vi "Intake State Controller.vi"(0 "Intake State":enum16{"Cone", "Cube", "Cube Handoff", "Stow"}(ring)=enum."Stow") -> ()   [LabVIEW 2020]
uses:
  <vilib>/Rock Robotics/WPI/Solenoid/WPI_SolenoidValue.ctl
  <vilib>/Rock Robotics/WPI/ThirdParty/REV Robotics/REVLib/Typedef/Spark MAX Control Type.ctl
  <vilib>/Rock Robotics/WPI/Solenoid/WPI_SolenoidSetEnum.vi
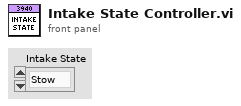
[diagram p1: front panel]
types:
  T1 = typedef "WPI_SolenoidDevRef.ctl" = cluster{"DevStatus":errorcluster, "Pneumatics Control Module":u8, "Forward Solenoid Channel":T2, "Reverse Solenoid Channel":T2}
  T2 = typedef "WPI_SolenoidChannel.ctl" = enum8{"Solenoid 0", "Solenoid 1", "Solenoid 2", "Solenoid 3", "Solenoid 4", "Solenoid 5", "Solenoid 6", "Solenoid 7", "Solenoid 8", "Solenoid 9", "Solenoid 10", "Solenoid 11", "Solenoid 12", "Solenoid 13", "Solenoid 14", "Solenoid 15", "Invalid"}
  T3 = typedef "WPI_MotorControlDeviceRef.ctl" = cluster{"DeviceStatus":errorcluster, "Type":T4, "PWM":cluster{"PWM Channel":T5, "DeadBand":T6}, "CAN":cluster{"Device Number":u8, "SetOutput VI Ref":variant, "GetOutput VI Ref":variant, "Enable VI Ref":variant, "Disable VI Ref":variant, "Data":variant}, "Invert":bool, "DIO PWM":cluster{"PWM \"Enable\" Channel":T5, "DIOChannel":T7, "PWM Rate":dbl}}
  T4 = typedef "WPI_MotorControlType.ctl" = enum16{"PWM", "CAN", "DIO PWM"}
  T5 = typedef "FPGA_DIOPWMChannel.ctl" = enum8{"PWM 0", "PWM 1", "PWM 2", "PWM 3", "PWM 4", "PWM 5", "PWM 6", "PWM 7", "PWM 8", "PWM 9", "PWM MXP 0", "PWM MXP 1", "PWM MXP 2", "PWM MXP 3", "PWM MXP 4", "PWM MXP 5", "PWM MXP 6", "PWM MXP 7", "PWM MXP 8", "PWM MXP 9", "Invalid"}
  T6 = typedef "WPI_PWMDeadband.ctl" = cluster{"Name":string, "maxPositivePwm":i32, "minPositivePwm":i32, "centerPwm":i32, "maxNegativePwm":i32, "minNegativePwm":i32, "angularRange":u16}
  T7 = typedef "FPGA_DIOChannel.ctl" = enum8{"DIO 0", "DIO 1", "DIO 2", "DIO 3", "DIO 4", "DIO 5", "DIO 6", "DIO 7", "DIO 8", "DIO 9", "DIO MXP 0", "DIO MXP 1", "DIO MXP 2", "DIO MXP 3", "DIO MXP 4", "DIO MXP 5", "DIO MXP 6", "DIO MXP 7", "DIO MXP 8", "DIO MXP 9", "DIO MXP 10", "DIO MXP 11", "DIO MXP 12", "DIO MXP 13", "DIO MXP 14", "DIO MXP 15", "SPI Port CS1", "SPI Port CS2", "SPI Port CS3", "SPI Port MISO", "SPI Port MOSI", "Invalid"}
  T8 = typedef "WPI_SolenoidValue.ctl" = enum16{"Off", "On", "Forward", "Reverse"}
  T9 = typedef "Spark MAX Control Type.ctl" = enum16{"Percent VBus", "Voltage", "Velocity", "Position", "Smart Motion", "Current", "Smart Velocity"}
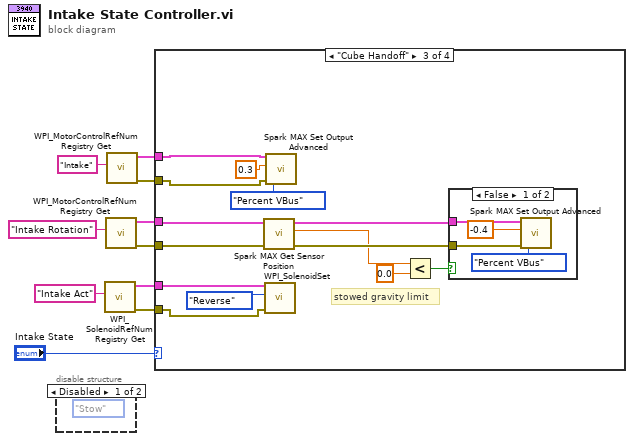
[diagram p0: block diagram]
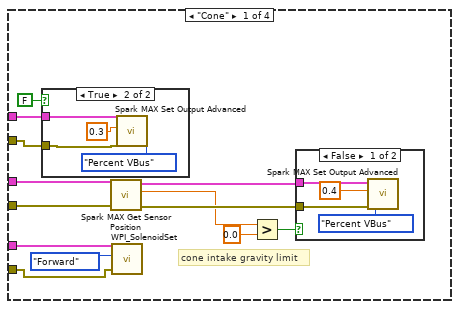
[diagram p3: hidden frame]
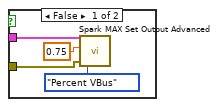
[diagram p4: hidden frame]
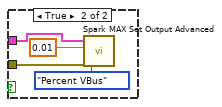
[diagram p5: hidden frame]
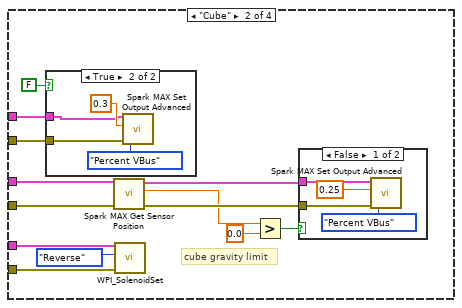
[diagram p6: hidden frame]
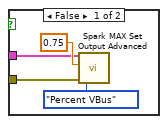
[diagram p7: hidden frame]
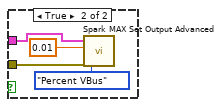
[diagram p8: hidden frame]
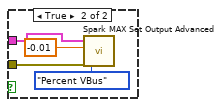
[diagram p9: hidden frame]
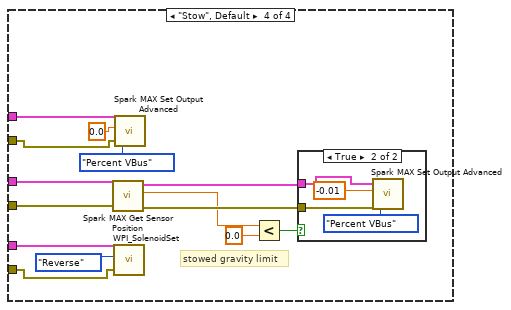
[diagram p10: hidden frame]
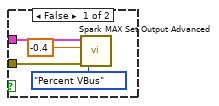
[diagram p11: hidden frame]
diagram:
  n1 = disable-structure shown="Disabled" {
    frame Disabled {
      (unwired) enum16{"Cone", "Cube", "Cube Handoff", "Stow"}."Stow"
    }
    frame Enabled {
    }
  }
  n2 = call <vilib>:"WPI_SolenoidRefNum Registry Get.vi"("refnum name"="Intake Act") -> ("error out"=w9:errorcluster, "SolenoidDevRef"=w10:T1)  [unwired: 9 in]
  n3 = call <vilib>:"WPI_MotorControlRefNum Registry Get.vi"("refnum name"="Intake Rotation") -> ("error out"=w5:errorcluster, "MotorControlDevRef"=w6:T3)  [unwired: 9 in]
  n4 = call <vilib>:"WPI_MotorControlRefNum Registry Get.vi"("refnum name"="Intake") -> ("error out"=w3:errorcluster, "MotorControlDevRef"=w4:T3)  [unwired: 9 in]
  n5 = case shown="\"Cube Handoff\"" "Intake State" {
    tunnel: w10 -> [w17 w42 w78 w92]
    tunnel: w9 -> [w16 w41 w77 w91]
    tunnel: w6 -> [w14 w44 w74 w94]
    tunnel: w5 -> [w15 w43 w73 w93]
    tunnel: w4 -> [w13 w46 w79 w96]
    tunnel: w3 -> [w12 w45 w69 w95]
    frame "Cone" {
      # "cone intake gravity limit"
      n6 = case shown="True" FALSE {
        tunnel: w13 -> [w25 w30]
        tunnel: w12 -> [w24 w29]
        frame False {
          n7 = call <vilib>:"Spark MAX Set Output Advanced.vi"("error in (no error)"=w24, "Control Mode"=Spark_MAX_Control_Type."Percent VBus", "Setpoint"=0.75, "MotorControlDevRef"=w25) -> ()  [unwired: 6 in, 2 out]
        }
        frame True {
          n8 = call <vilib>:"Spark MAX Set Output Advanced.vi"("error in (no error)"=w29, "Control Mode"=Spark_MAX_Control_Type."Percent VBus", "Setpoint"=0.3, "MotorControlDevRef"=w30) -> ()  [unwired: 6 in, 2 out]
        }
      }
      n9 = call <vilib>:"Spark MAX Get Sensor Position.vi"("error in (no error)"=w15, "MotorControlDevRef in"=w14) -> ("error out"=w21:errorcluster, "Sensor Position"=w19:dbl, "MotorControlDevRef out"=w22:T3)  [unwired: 6 in, 1 out]
      n10 = call-poly <vilib>:"WPI_SolenoidSet.vi"("error in (no error)"=w16, "Value"=WPI_SolenoidValue."Forward", "SolenoidDevRef"=w17) -> ()  [unwired: 7 in, 2 out]
      n11 = Greater?(x=w19, y=0.0) -> (0:w20:bool)
      n12 = case shown="False" w20 {
        tunnel: w22 -> [w33 w37]
        tunnel: w21 -> [w32 w36]
        frame False {
          n13 = call <vilib>:"Spark MAX Set Output Advanced.vi"("error in (no error)"=w32, "Control Mode"=Spark_MAX_Control_Type."Percent VBus", "Setpoint"=0.4, "MotorControlDevRef"=w33) -> ()  [unwired: 6 in, 2 out]
        }
        frame True {
          n14 = call <vilib>:"Spark MAX Set Output Advanced.vi"("error in (no error)"=w36, "Control Mode"=Spark_MAX_Control_Type."Percent VBus", "Setpoint"=0.01, "MotorControlDevRef"=w37) -> ()  [unwired: 6 in, 2 out]
        }
      }
    }
    frame "Cube" {
      # "cube gravity limit"
      n15 = case shown="True" FALSE {
        tunnel: w46 -> [w54 w58]
        tunnel: w45 -> [w53 w57]
        frame False {
          n16 = call <vilib>:"Spark MAX Set Output Advanced.vi"("error in (no error)"=w53, "Control Mode"=Spark_MAX_Control_Type."Percent VBus", "Setpoint"=0.75, "MotorControlDevRef"=w54) -> ()  [unwired: 6 in, 2 out]
        }
        frame True {
          n17 = call <vilib>:"Spark MAX Set Output Advanced.vi"("error in (no error)"=w57, "Control Mode"=Spark_MAX_Control_Type."Percent VBus", "Setpoint"=0.3, "MotorControlDevRef"=w58) -> ()  [unwired: 6 in, 2 out]
        }
      }
      n18 = call <vilib>:"Spark MAX Get Sensor Position.vi"("error in (no error)"=w43, "MotorControlDevRef in"=w44) -> ("error out"=w50:errorcluster, "Sensor Position"=w48:dbl, "MotorControlDevRef out"=w51:T3)  [unwired: 6 in, 1 out]
      n19 = call-poly <vilib>:"WPI_SolenoidSet.vi"("error in (no error)"=w41, "Value"=WPI_SolenoidValue."Reverse", "SolenoidDevRef"=w42) -> ()  [unwired: 7 in, 2 out]
      n20 = Greater?(x=w48, y=0.0) -> (0:w49:bool)
      n21 = case shown="False" w49 {
        tunnel: w51 -> [w62 w66]
        tunnel: w50 -> [w61 w65]
        frame False {
          n22 = call <vilib>:"Spark MAX Set Output Advanced.vi"("error in (no error)"=w61, "Control Mode"=Spark_MAX_Control_Type."Percent VBus", "Setpoint"=0.25, "MotorControlDevRef"=w62) -> ()  [unwired: 6 in, 2 out]
        }
        frame True {
          n23 = call <vilib>:"Spark MAX Set Output Advanced.vi"("error in (no error)"=w65, "Control Mode"=Spark_MAX_Control_Type."Percent VBus", "Setpoint"=0.01, "MotorControlDevRef"=w66) -> ()  [unwired: 6 in, 2 out]
        }
      }
    }
    frame "Cube Handoff" {
      # "stowed gravity limit"
      n24 = call <vilib>:"Spark MAX Get Sensor Position.vi"("error in (no error)"=w73, "MotorControlDevRef in"=w74) -> ("error out"=w75:errorcluster, "Sensor Position"=w71:dbl, "MotorControlDevRef out"=w76:T3)  [unwired: 6 in, 1 out]
      n25 = call-poly <vilib>:"WPI_SolenoidSet.vi"("error in (no error)"=w77, "Value"=WPI_SolenoidValue."Reverse", "SolenoidDevRef"=w78) -> ()  [unwired: 7 in, 2 out]
      n26 = call <vilib>:"Spark MAX Set Output Advanced.vi"("error in (no error)"=w69, "Control Mode"=Spark_MAX_Control_Type."Percent VBus", "Setpoint"=0.3, "MotorControlDevRef"=w79) -> ()  [unwired: 6 in, 2 out]
      n27 = Less?(x=w71, y=0.0) -> (x < y?=w72:bool)
      n28 = case shown="False" w72 {
        tunnel: w76 -> [w84 w88]
        tunnel: w75 -> [w83 w87]
        frame False {
          n29 = call <vilib>:"Spark MAX Set Output Advanced.vi"("error in (no error)"=w83, "Control Mode"=Spark_MAX_Control_Type."Percent VBus", "Setpoint"=-0.4, "MotorControlDevRef"=w84) -> ()  [unwired: 6 in, 2 out]
        }
        frame True {
          n30 = call <vilib>:"Spark MAX Set Output Advanced.vi"("error in (no error)"=w87, "Control Mode"=Spark_MAX_Control_Type."Percent VBus", "Setpoint"=-0.01, "MotorControlDevRef"=w88) -> ()  [unwired: 6 in, 2 out]
        }
      }
    }
    frame "Stow", Default {
      # "stowed gravity limit"
      n31 = call <vilib>:"Spark MAX Get Sensor Position.vi"("error in (no error)"=w93, "MotorControlDevRef in"=w94) -> ("error out"=w100:errorcluster, "Sensor Position"=w98:dbl, "MotorControlDevRef out"=w101:T3)  [unwired: 6 in, 1 out]
      n32 = call-poly <vilib>:"WPI_SolenoidSet.vi"("error in (no error)"=w91, "Value"=WPI_SolenoidValue."Reverse", "SolenoidDevRef"=w92) -> ()  [unwired: 7 in, 2 out]
      n33 = call <vilib>:"Spark MAX Set Output Advanced.vi"("error in (no error)"=w95, "Control Mode"=Spark_MAX_Control_Type."Percent VBus", "Setpoint"=0.0, "MotorControlDevRef"=w96) -> ()  [unwired: 6 in, 2 out]
      n34 = Less?(x=w98, y=0.0) -> (x < y?=w99:bool)
      n35 = case shown="True" w99 {
        tunnel: w101 -> [w106 w110]
        tunnel: w100 -> [w105 w109]
        frame False {
          n36 = call <vilib>:"Spark MAX Set Output Advanced.vi"("error in (no error)"=w105, "Control Mode"=Spark_MAX_Control_Type."Percent VBus", "Setpoint"=-0.4, "MotorControlDevRef"=w106) -> ()  [unwired: 6 in, 2 out]
        }
        frame True {
          n37 = call <vilib>:"Spark MAX Set Output Advanced.vi"("error in (no error)"=w109, "Control Mode"=Spark_MAX_Control_Type."Percent VBus", "Setpoint"=-0.01, "MotorControlDevRef"=w110) -> ()  [unwired: 6 in, 2 out]
        }
      }
    }
  }
